vi "testy 3dconnectionn.vi"() -> ()   [LabVIEW 2015]
uses:
  <vilib>/picture/3D Picture Control/Object/Create Object (drawable).vi
  <vilib>/Utility/inputDevices.llb/joystickAcquire.vi
  <vilib>/Utility/inputDevices.llb/closeJoystick.vi
  <vilib>/picture/3D Picture Control/NI_3D Picture Control.lvlib
panel:
  in  "Color":T1={"Red"=1.0, "Green"=0.0, "Blue"=0.0, "Alpha"=1.0}
  in  "Numeric":dbl=1.0 format="%#_13g"
  out "3D Picture":refnum<vi>(3d-picture)
  in  "device index":i32
  out "direction info":T2
  out "button info":T3
  out "axis info":T4
  in  "stop":bool
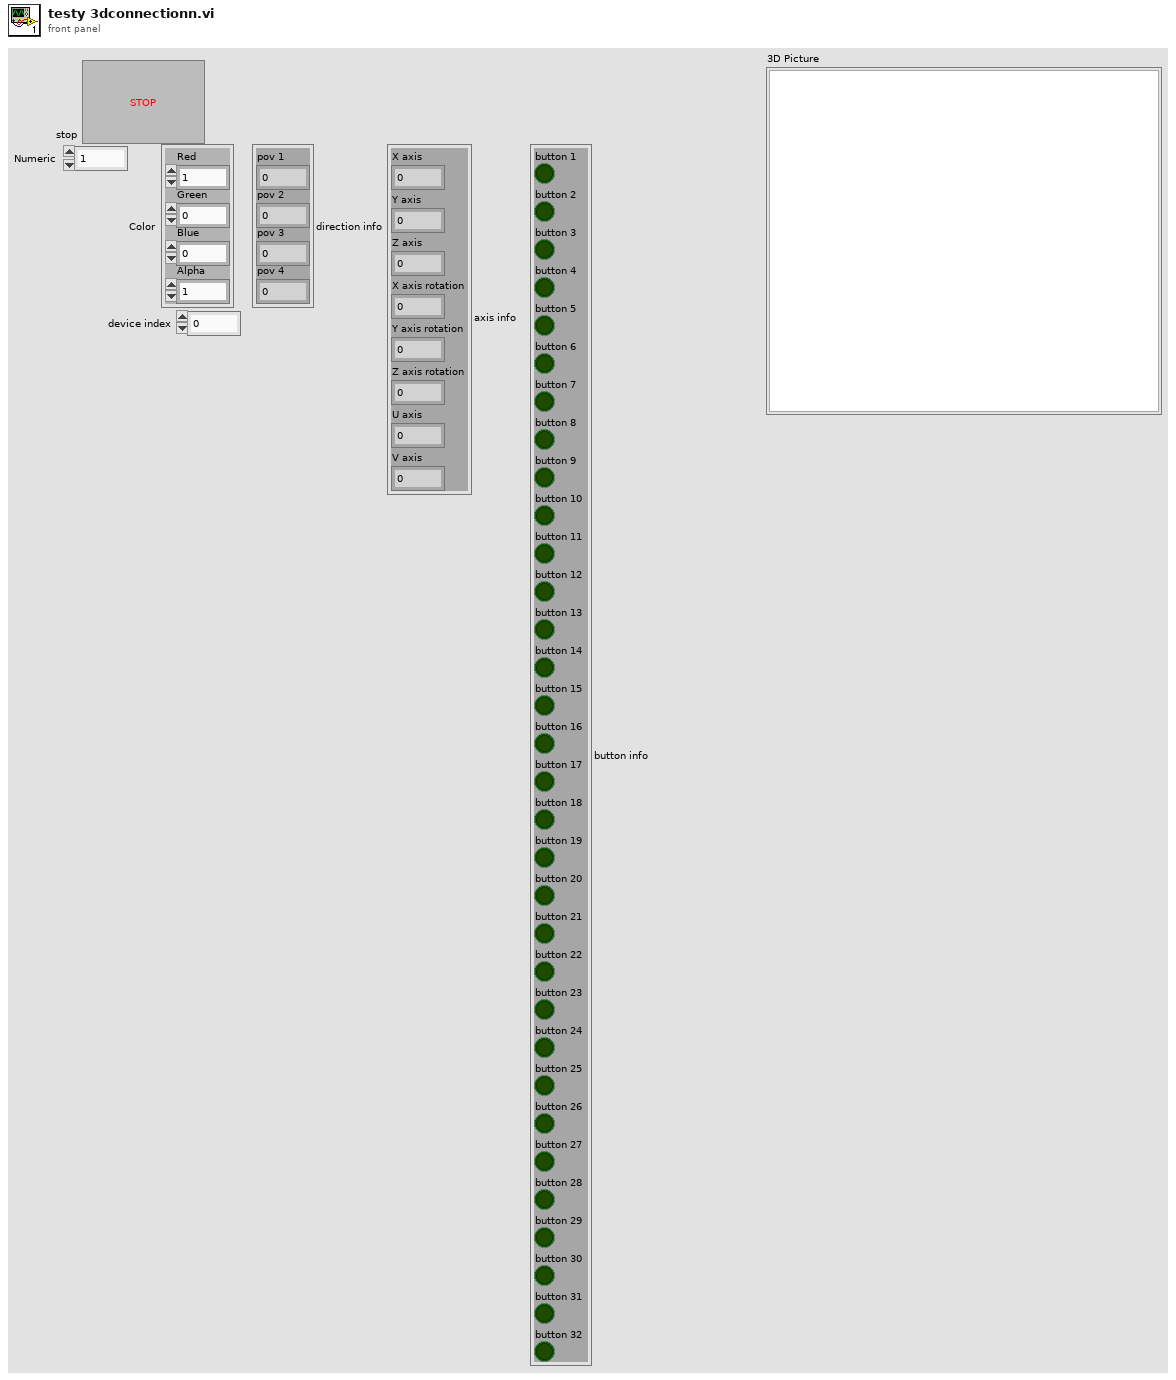
[diagram p1: front panel]
types:
  T1 = cluster{"Red":sgl, "Green":sgl, "Blue":sgl, "Alpha":sgl}
  T2 = cluster{"pov 1":i32, "pov 2":i32, "pov 3":i32, "pov 4":i32}
  T3 = cluster{"button 1":bool, "button 2":bool, "button 3":bool, "button 4":bool, "button 5":bool, "button 6":bool, "button 7":bool, "button 8":bool, "button 9":bool, "button 10":bool, "button 11":bool, "button 12":bool, "button 13":bool, "button 14":bool, "button 15":bool, "button 16":bool, "button 17":bool, "button 18":bool, "button 19":bool, "button 20":bool, "button 21":bool, "button 22":bool, "button 23":bool, "button 24":bool, "button 25":bool, "button 26":bool, "button 27":bool, "button 28":bool, "button 29":bool, "button 30":bool, "button 31":bool, "button 32":bool}
  T4 = cluster{"X axis":i32, "Y axis":i32, "Z axis":i32, "X axis rotation":i32, "Y axis rotation":i32, "Z axis rotation":i32, "U axis":i32, "V axis":i32}
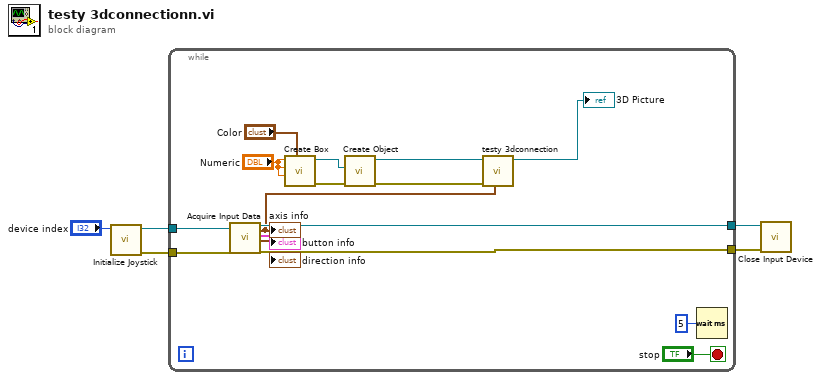
[diagram p0: block diagram]
diagram:
  n1 = call <vilib>:"Initialize Joystick.vi"("device index"="device index") -> ("error out"=w4:errorcluster, "device ID"=w5:refnum<k1>)  [unwired: 9 in]
  n2 = while {
    tunnel: w5 -> [w19]
    tunnel: w4 -> [w18]
    tunnel: [w7] -> w3
    tunnel: [w17] -> w2
    stop <- "stop" stop-if-true
    n3 = call-poly <vilib>:"Acquire Input Data.vi"("device ID"=w19, "error in (no error)"=w18) -> ("device ID"=w7:refnum<k1>, "axis info"=w6:T4, "button info"=→"button info":T3, "direction info"=→"direction info":T2, "error out"=w17:errorcluster)  [unwired: 13 in]
    "axis info" <- w6
    n4 = call <vilib>:"Create Box.vi"("Color"="Color", "Length Z"="Numeric", "Length Y"="Numeric", "Length X"="Numeric") -> ("error out"=w11:errorcluster, "New Box Refnum"=w12:refnum<vi>)  [unwired: 6 in]
    n5 = call-poly <vilib>:"Create Object.vi"("error in (no error)"=w11, "Geometry"=w12) -> ("error out"=w9:errorcluster, "Scene:New Object"=w10:refnum<vi>)  [unwired: 8 in]
    n6 = call "testy 3dconnection.vi"("axis info 2"=w6, "error in (no error)"=w9, "SceneObject in"=w10) -> ("SceneObject out"=→"3D Picture":refnum<vi>)  [unwired: 8 in]
    n7 = Wait (ms)(milliseconds to wait=u32 5) -> ()  [unwired: 1 out]
  }
  n8 = call-poly <vilib>:"Close Input Device.vi"("error in (no error)"=w2, "device ID"=w3) -> ()  [unwired: 8 in, 1 out]
